vi "Status Preset.vi"(0 "VISA resource name":refnum<visa-resource-name>, 11 "error in (no error)":errorcluster) -> (4 "VISA resource name out":refnum<visa-resource-name>, 15 "error out":errorcluster)   [LabVIEW 2018, in "XP Power PLS600.lvlib"]
doc: "Sets the value of all the enable registers (operation and questionable) to 0 (ALL disabled).\n\nThis only affects the enable registers. It does not affect either the “status byte” or the “standard event status” as defined by IEEE 488.2. This does not clear any of the event registers or any item from the error/event queue. The *CLS command is used to clear all event registers and queues in the device status-reporting mechanism. For the SCPI mandatory status data structures, this command sets the enable registers to 0’s."
uses:
  XP Power PLS600.lvlib
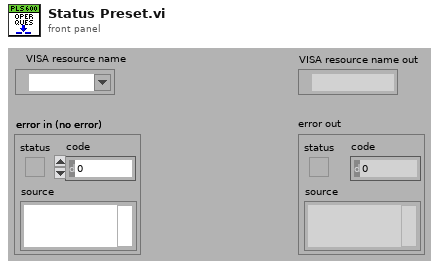
[diagram p1: front panel]
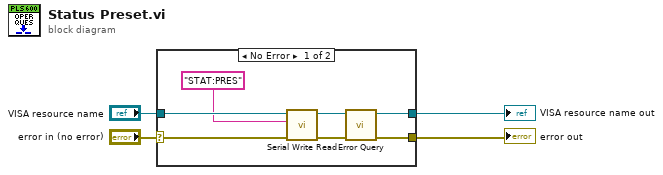
[diagram p0: block diagram]
diagram:
  n1 = case shown="No Error" "error in (no error)" {
    selector: "error in (no error)" -> [w9 w12]
    tunnel: "VISA resource name" -> [w10 w13]
    tunnel: [w6 w13] -> w3
    tunnel: [w7 w12] -> w2
    frame No Error {
      n2 = call "Serial Write Read.vi"("error in (no error)"=w9, "Write Buffer"="STAT:PRES", "VISA resource name"=w10) -> ("error out"=w8:errorcluster, "VISA resource name out"=w11:refnum<visa-resource-name>)  [unwired: 6 in, 1 out]
      n3 = call "Error Query.vi"("error in (no error)"=w8, "VISA resource name"=w11) -> ("error out"=w7:errorcluster, "VISA resource name out"=w6:refnum<visa-resource-name>)  [unwired: 6 in, 2 out]
    }
    frame Error {
    }
  }
  "error out" <- w2
  "VISA resource name out" <- w3
